vi "Generate ID.vi"() -> (2 "Unique ID":i32)   [LabVIEW 2015, in "Formics.lvclass"]
uses:
  Formics.lvclass
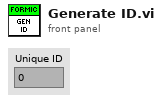
[diagram p1: front panel]
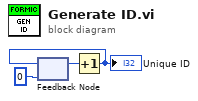
[diagram p0: block diagram]
diagram:
  n1 = feedback #1(0) -> (w2:i32)
  n2 = Increment(x=w2) -> (x+1=w1:i32)
  "Unique ID" <- w1
  n3 = feedback-in #1(w1) -> ()
